vi "motor.vi"() -> ()   [LabVIEW 2014]
uses:
  <vilib>/LabVIEW Interface for Arduino/Type Defs/Pin Mode.ctl
  <vilib>/LabVIEW Interface for Arduino/LabVIEW Interface for Arduino.lvlib
panel:
  in  "VISA resource":refnum<visa-resource-name>
  out "Speed":dbl(knob) scale=0.0..100.0
  in  "Dial":dbl(knob) scale=0.0..255.0
  in  "INPUT 2":bool
  in  "INPUT 1":bool
  in  "stop":bool
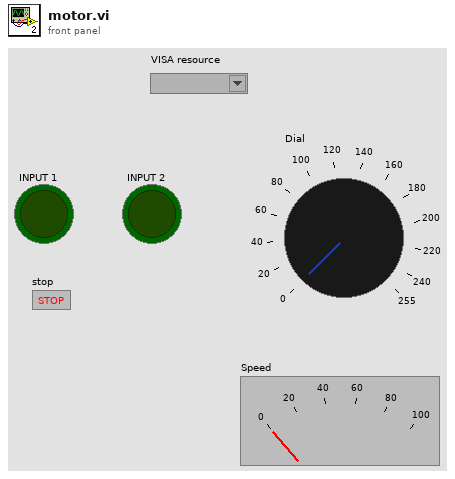
[diagram p1: front panel]
types:
  T1 = typedef "LabVIEW Interface for Arduino.lvlib/Arduino Resource.ctl" = cluster{"VISA resource":refnum<visa-resource-name>, "Board Type":T2, "Connection Type":enum8{"USB / Serial"}, "Bytes Per Packet (15)":u8}
  T2 = typedef "LabVIEW Interface for Arduino.lvlib/Board Type.ctl" = enum16{"Uno", "Dimuelanove w/Atmega 328", "Mega 2560"}
  T3 = typedef "LabVIEW Interface for Arduino.lvlib/Pin Mode.ctl" = enum8{"Input", "Output"}
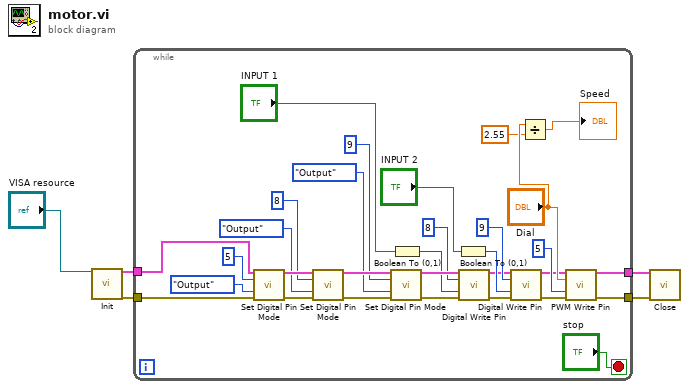
[diagram p0: block diagram]
diagram:
  n1 = call <vilib>:"Init.vi"("VISA resource"="VISA resource") -> ("Arduino Resource"=w3:T1, "error out"=w2:errorcluster)  [unwired: 17 in]
  n2 = while {
    tunnel: w3 -> [w36]
    tunnel: w2 -> [w35]
    tunnel: [w11] -> w5
    tunnel: [w10] -> w4
    stop <- "stop" stop-if-true
    n3 = call <vilib>:"Set Digital Pin Mode.vi"("Arduino Resource"=w36, "Digital I/O Pin"=u8 5, "Pin Mode (Input)"=Pin_Mode."Output", "error in"=w35) -> ("Arduino Resource"=w31:T1, "error out"=w30:errorcluster)  [unwired: 10 in]
    n4 = call <vilib>:"Set Digital Pin Mode.vi"("Arduino Resource"=w31, "Digital I/O Pin"=u8 8, "Pin Mode (Input)"=Pin_Mode."Output", "error in"=w30) -> ("Arduino Resource"=w27:T1, "error out"=w26:errorcluster)  [unwired: 10 in]
    n5 = call <vilib>:"Set Digital Pin Mode.vi"("Arduino Resource"=w27, "Digital I/O Pin"=u8 9, "Pin Mode (Input)"=Pin_Mode."Output", "error in"=w26) -> ("Arduino Resource"=w23:T1, "error out"=w22:errorcluster)  [unwired: 10 in]
    n6 = Boolean To (0,1)(Boolean="INPUT 1") -> (0, 1=w19:i16)
    n7 = Boolean To (0,1)(Boolean="INPUT 2") -> (0, 1=w16:i16)
    n8 = call <vilib>:"Digital Write Pin.vi"("Arduino Resource"=w23, "Digital I/O Pin (0)"=u8 8, "Value (0)"=w19, "error in"=w22) -> ("Arduino Resource"=w15:T1, "error out"=w14:errorcluster)  [unwired: 10 in]
    n9 = call <vilib>:"Digital Write Pin.vi"("Arduino Resource"=w15, "Digital I/O Pin (0)"=u8 9, "Value (0)"=w16, "error in"=w14) -> ("Arduino Resource"=w6:T1, "error out"=w13:errorcluster)  [unwired: 10 in]
    n10 = Divide(x="Dial", y=2.55) -> (x/y=→"Speed":dbl)
    n11 = call <vilib>:"PWM Write Pin.vi"("Arduino Resource"=w6, "Duty Cycle (0 - 255)"="Dial", "PWM Pin (3)"=u8 5, "error in"=w13) -> ("Arduino Resource"=w11:T1, "error out"=w10:errorcluster)  [unwired: 10 in]
  }
  n12 = call <vilib>:"Close.vi"("Arduino Resource"=w5, "error in"=w4) -> ()  [unwired: 13 in, 1 out]
